vi "Error Strings Global Internal.vi"() -> ()   [LabVIEW 2021, in "InstrumentStudio Plug-In Editor.lvlib"]
uses:
  InstrumentStudio Plug-In Editor.lvlib
panel:
  out "5002":string="Could not find the InstrumentStudio plug-in library template at the provided path: '%s'."
  out "5001":string="The project folder path '%s' is empty or invalid."
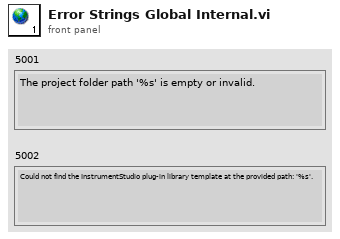
[diagram p1: front panel]
diagram:
